vi "Generate Code.vi"(8 "error in":errorcluster, 11 "node in":refnum<class "RIO Target.lvclass">) -> (0 "error out":errorcluster)   [LabVIEW 2014, in "RIO Target.lvclass"]
uses:
  RIO Target.lvclass
  System.Windows.Forms
  Scripting/Initialization Scripting/State Machine/Controls/Input Paths.ctl
  Scripting/Initialization Scripting/State Machine/Top Level State Machine.vi
  Scripting/Initialization Scripting/Initialization and IO Node Scripting.lvlib
panel:
  in  "Status":string
  in  "ProgressBar":refnum<k24>(container)
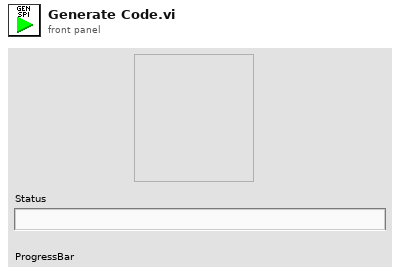
[diagram p1: front panel]
types:
  T1 = typedef "Input Paths.ctl" = cluster{"Golden Template (Source) - (make relative)":path, "Destination Generated Code (make relative)":path, "LabVIEW Project to Script":path, "VI to which to Add Engines and IO Nodes":path}
  T2 = typedef "Initialization and IO Node Scripting.lvlib/Bus Information.ctl" = cluster{"Devices":T3[], "Pin Information":T4, "Replacement VI for DLU":path}
  T3 = typedef "Device Information.ctl" = cluster{"Number of Channels":i32, "Device Alias":string, "Device Icon Name":string[]}
  T4 = typedef "Pin Information.ctl" = cluster{"List of IO Names":string[], "List of Enable Lines":string[]}
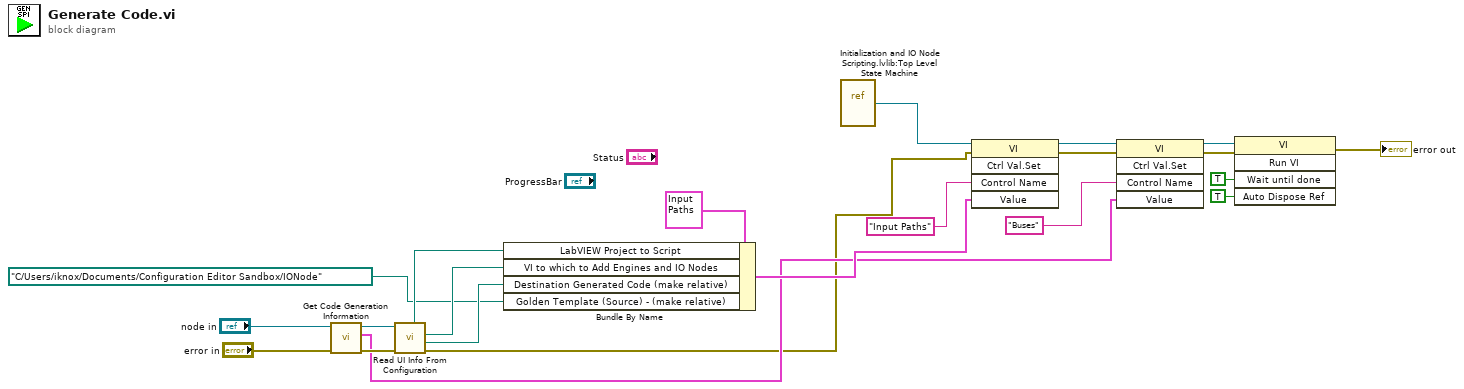
[diagram p0: block diagram]
diagram:
  n1 = call "Get Code Generation Information.vi"("error in (no error)"="error in", "RIO Target in"="node in") -> ("error out"=w19:errorcluster, "Bus Information Array"=w7:T2[], "RIO Target out"=w17:refnum<class "RIO Target.lvclass">)  [unwired: 7 in]
  n2 = call "Read UI Info From Configuration.vi"("error in (no error)"=w19, "node in"=w17) -> ("error out"=w2:errorcluster, "Destination Path"=w20:path, "VI to Place Engines and IO Nodes"=w21:path, "Target Project Path"=w22:path)  [unwired: 5 in, 1 out]
  n3 = Bundle By Name(cluster=T1 {"Golden Template (Source) - (make relative)"=path "C:/Users/iknox/Documents/Configuration Editor Sandbox/IONode", "Destination Generated Code (make relative)"=path "C:/Users/iknox/Desktop/Test", "LabVIEW Project to Script"=path "C:/Users/iknox/Desktop/Untitled Project 1.lvproj", "VI to which to Add Engines and IO Nodes"=path "C:/Users/iknox/Desktop/Untitled 3.vi"} ("Input Paths"), "LabVIEW Project to Script"=w22, "VI to which to Add Engines and IO Nodes"=w21, "Destination Generated Code (make relative)"=w20, "Golden Template (Source) - (make relative)"=path "C:/Users/iknox/Documents/Configuration Editor Sandbox/IONode" ("Golden Template Source Path (testing only)")) -> (w8:T1)
  n4 = vi-ref "Initialization and IO Node Scripting.lvlib:Top Level State Machine.vi"() -> (w1:refnum<vi>)
  n5 = invoke class="VI" method="Ctrl Val.Set"(reference=w1, error in=w2, "Control Name"="Input Paths", "Value"=w8) -> (reference out=w11:refnum<vi>, error out=w6:errorcluster)  [unwired: 1 in, 3 out]
  n6 = invoke class="VI" method="Ctrl Val.Set"(reference=w11, error in=w6, "Control Name"="Buses", "Value"=w7) -> (reference out=w5:refnum<vi>, error out=w3:errorcluster)  [unwired: 1 in, 3 out]
  n7 = invoke class="VI" method="Run VI"(reference=w5, error in=w3, "Wait until done"=TRUE ("Wait Until Done"), "Auto Dispose Ref"=TRUE ("Auto Dispose Reference")) -> (error out=→"error out":errorcluster)  [unwired: 1 in, 4 out]
